vi "Control de velocidad serial.vi"() -> ()   [LabVIEW 2019]
uses:
  <vilib>/Instr/_visa.llb/VISA Configure Serial Port (Instr).vi
panel:
  out "Velocidad (indicador)":dbl
  in  "Arranque / Paro":bool
  in  "Sentido de giro":bool
  out "error out":errorcluster
  in  "stop":bool
  in  "VISA resource name":refnum<visa-resource-name>
  in  "Velocidad":dbl(slide) scale=500.0..1000.0
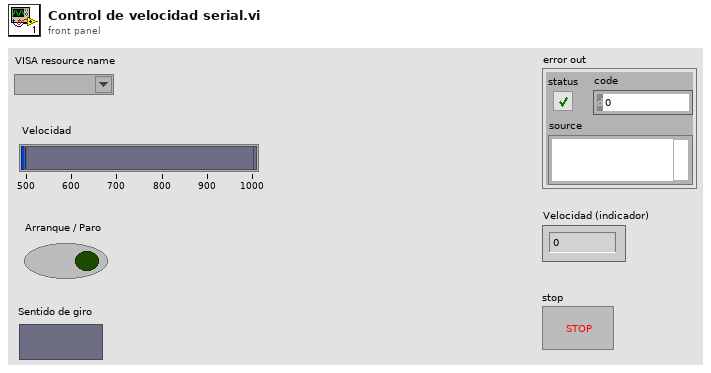
[diagram p1: front panel]
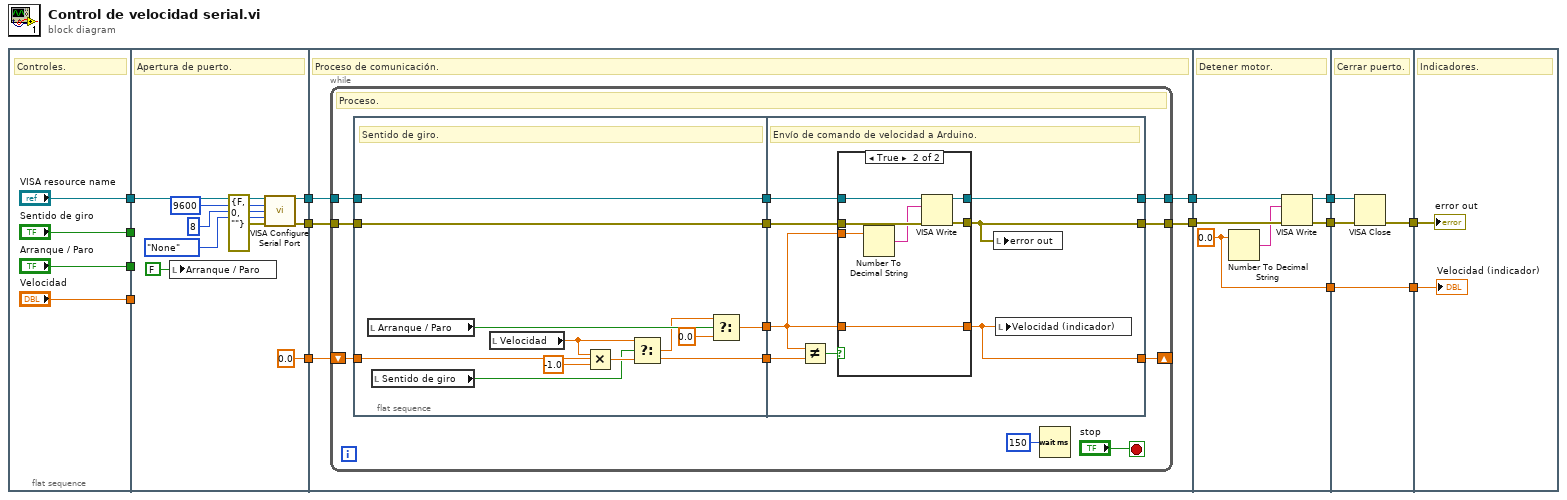
[diagram p0: block diagram]
diagram:
  n1 = flat-sequence {
    tunnel: ["VISA resource name"] -> w14
    tunnel: ["Sentido de giro"] -> w13
    tunnel: ["Arranque / Paro"] -> w9
    tunnel: ["Velocidad"] -> w8
    tunnel: w14 -> [w26]
    tunnel: w13 -> [_]
    tunnel: [w25] -> w12
    tunnel: [w24] -> w11
    tunnel: [0.0 ("Slide")] -> w10
    tunnel: w9 -> [_]
    tunnel: w8 -> [_]
    tunnel: [w28] -> w5
    tunnel: [w29] -> w3
    tunnel: w12 -> [w31]
    tunnel: w11 -> [w30]
    tunnel: w10 -> [w32]
    tunnel: w5 -> [w77]
    tunnel: [w76] -> w4
    tunnel: w3 -> [w79]
    tunnel: [w78] -> w2
    tunnel: [w74] -> w1
    tunnel: w4 -> [w82]
    tunnel: w2 -> [w83]
    tunnel: [w81] -> w7
    tunnel: [w80] -> w6
    tunnel: w1 -> [w80]
    tunnel: w7 -> [w85]
    tunnel: w6 -> [w84]
    frame #0 {
      # "Controles."
    }
    frame #1 {
      # "Apertura de puerto."
      n2 = local write "Arranque / Paro"(FALSE ("Arranque / Paro")) -> ()
      n3 = call-poly "VISA Configure Serial Port"("VISA resource name"=w26, "baud rate (9600)"=u32 9600, "data bits (8)"=u16 8, "parity (0:none)"=enum16{"None", "Odd", "Even", "Mark", "Space"}."None", "error in (no error)"=errorcluster {"status"=FALSE, "code"=0, "source"=""}) -> ("VISA resource name out"=w25:refnum<visa-resource-name>, "error out"=w24:errorcluster)  [unwired: 9 in]
    }
    frame #2 {
      # "Proceso de comunicación."
      n4 = while {
        shift-right: [w33] -> _
        shift-left: w32 -> [w41]
        tunnel: w31 -> [w39]
        tunnel: w30 -> [w38]
        tunnel: [w35] -> w29
        tunnel: [w34] -> w28
        stop <- "stop" stop-if-true
        # "Proceso."
        n5 = flat-sequence {
          tunnel: [w46] -> w42
          tunnel: w41 -> [w52]
          tunnel: [w52] -> w40
          tunnel: w39 -> [w51]
          tunnel: w38 -> [w50]
          tunnel: [w51] -> w37
          tunnel: [w50] -> w36
          tunnel: w42 -> [w58]
          tunnel: w40 -> [w63]
          tunnel: w37 -> [w62]
          tunnel: w36 -> [w61]
          tunnel: [w60] -> w35
          tunnel: [w57] -> w34
          tunnel: [w56] -> w33
          frame #0 {
            # "Sentido de giro."
            n6 = local read "Arranque / Paro"() -> (w49:bool)
            n7 = local read "Sentido de giro"() -> (w45:bool)
            n8 = local read "Velocidad"() -> (w53:dbl)
            n9 = Multiply(x=w53, y=-1.0) -> (x*y=w54:dbl)
            n10 = Select(t=w53, s=w45, f=w54) -> (s? t:f=w47:dbl)
            n11 = Select(t=w47, s=w49, f=0.0) -> (s? t:f=w46:dbl)
          }
          frame #1 {
            # "Envío de comando de velocidad a Arduino."
            n12 = Not Equal?(x=w58, y=w63) -> (x != y?=w59:bool)
            n13 = case shown="True" w59 {
              tunnel: w62 -> [w66 w73]
              tunnel: w61 -> [w65 w72]
              tunnel: [w66 w71] -> w60
              tunnel: [w65 w69] -> w57
              tunnel: w58 -> [_ w68]
              tunnel: w58 -> [w64 w67]
              tunnel: [w64 w67] -> w56
              frame False {
              }
              frame True {
                n14 = Number To Decimal String(number=w68) -> (decimal integer string=w70:string)  [unwired: 1 in]
                n15 = VISA Write(VISA resource name=w73, write buffer=w70, error in (no error)=w72) -> (VISA resource name out=w71:refnum<visa-resource-name>, error out=w69:errorcluster)  [unwired: 1 out]
              }
            }
            n16 = local write "error out"(w57) -> ()
            n17 = local write "Velocidad (indicador)"(w56) -> ()
          }
        }
        n18 = Wait (ms)(milliseconds to wait=u32 150) -> ()  [unwired: 1 out]
      }
    }
    frame #3 {
      w74 = 0.0 ("f")
      # "Detener motor."
      n19 = Number To Decimal String(number=w74) -> (decimal integer string=w75:string)  [unwired: 1 in]
      n20 = VISA Write(VISA resource name=w79, write buffer=w75, error in (no error)=w77) -> (VISA resource name out=w78:refnum<visa-resource-name>, error out=w76:errorcluster)  [unwired: 1 out]
    }
    frame #4 {
      # "Cerrar puerto."
      n21 = VISA Close(VISA resource name=w83, error in (no error)=w82) -> (error out=w81:errorcluster)
    }
    frame #5 {
      # "Indicadores."
      "error out" <- w85
      "Velocidad (indicador)" <- w84
    }
  }
